vi "macro_TrajectoryConstraint_MecaKine.vi"   [LabVIEW 2019, in "Trajectory_Library.lvlib"]
uses:
  Trajectory_Library.lvlib
types:
  T1 = typedef "Trajectory_Library.lvlib/TRANSLATION2D.ctl" = cluster{"X":dbl, "Y":dbl}
  T2 = typedef "Trajectory_Library.lvlib/MECA_DRIVE_KINEMATICS.ctl" = cluster{"FrontLeft":T1, "FrontRight":T1, "RearLeft":T1, "RearRight":T1, "InverseKinematics":T3, "ForwardKinematics":T3, "PrevCoR":T1}
  T3 = typedef "NI_Matrix.lvlib/RealMatrix.ctl" = dbl[][]
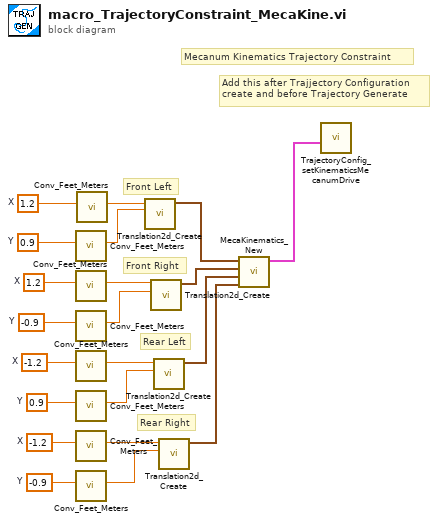
[diagram p0: block diagram]
diagram:
  w11 = -1.2  # X
  w10 = -0.9  # Y
  w13 = -1.2  # X
  w12 = 0.9  # Y
  w15 = 1.2  # X
  w14 = -0.9  # Y
  w17 = 1.2  # X
  w16 = 0.9  # Y
  # "Mecanum Kinematics Trajectory Constraint"
  # "Rear Right"
  # "Rear Left"
  # "Front Right"
  # "Front Left"
  # "Add this after Trajjectory Configuration\ncreate and before Trajectory Generate"
  n1 = call "Conv_Feet_Meters.vi"("Feet"=w16) -> ("Meters"=w8:dbl)  [unwired: 10 in]
  n2 = call "Conv_Feet_Meters.vi"("Feet"=w15) -> ("Meters"=w7:dbl)  [unwired: 10 in]
  n3 = call "Conv_Feet_Meters.vi"("Feet"=w14) -> ("Meters"=w6:dbl)  [unwired: 10 in]
  n4 = call "Conv_Feet_Meters.vi"("Feet"=w13) -> ("Meters"=w5:dbl)  [unwired: 10 in]
  n5 = call "Conv_Feet_Meters.vi"("Feet"=w12) -> ("Meters"=w4:dbl)  [unwired: 10 in]
  n6 = call "Conv_Feet_Meters.vi"("Feet"=w11) -> ("Meters"=w3:dbl)  [unwired: 10 in]
  n7 = call "Conv_Feet_Meters.vi"("Feet"=w10) -> ("Meters"=w2:dbl)  [unwired: 10 in]
  n8 = call "Conv_Feet_Meters.vi"("Feet"=w17) -> ("Meters"=w9:dbl)  [unwired: 10 in]
  n9 = call "Translation2d_Create.vi"("Y"=w8, "X"=w9) -> ("TRANSLATION"=w21:T1)  [unwired: 9 in]
  n10 = call "Translation2d_Create.vi"("Y"=w6, "X"=w7) -> ("TRANSLATION"=w20:T1)  [unwired: 9 in]
  n11 = call "Translation2d_Create.vi"("Y"=w4, "X"=w5) -> ("TRANSLATION"=w19:T1)  [unwired: 9 in]
  n12 = call "Translation2d_Create.vi"("Y"=w2, "X"=w3) -> ("TRANSLATION"=w18:T1)  [unwired: 9 in]
  n13 = call "MecaKinematics_New.vi"("RearRight"=w18, "RearLeft"=w19, "FrontRight"=w20, "FrontLeft"=w21) -> ("MECA_DRIVE_KINEMATICS"=w1:T2)  [unwired: 7 in]
  n14 = call "TrajectoryConfig_setKinematicsMecanumDrive.vi"("MECA_DRIVE_KINEMATICS"=w1) -> ()  [unwired: 10 in, 1 out]
